vi "DISP_WIND_TRAC_FEED.vi"(0 "VISA IN":refnum<visa-resource-name>, 1 "Trace":i32=1, 2 "Name":string, 5 "error in":errorcluster, 7 "Window":i32=1) -> (14 "VISA Out":refnum<visa-resource-name>, 19 "error out":errorcluster)   [LabVIEW 2018, in "PNA-X.lvlib"]
doc: "DISPlay:WINDow<wnum>:TRACe<tnum>:FEED <name> \n1595\n\n(Write-only) Creates a new trace <tnum> and associates (feeds) a measurement <name> to the \nspecified window<wnum>. This command should be executed immediately after creating a new \nmeasurement with CALC:PAR:DEF<name>,<parameter>. \nTo feed the same measurement to multiple traces, create another measurement with the same \n<name>,<parameter> using the CALC:PAR:DEF command. The analyzer will collect the data only \nonce. \nParameters \n<wnum> Any existing window number. If unspecified, value is set to 1. \n<tnum> Trace number to be created. Choose any Integer between 1 and 8 \n<name> Name of the measurement that was defined with \nCALC:PAR:DEF<name>,<parameter> \nExamples DISP:WIND:TRAC:FEED 'test' \ndisplay:window2:trace2:feed 'test' \nQuery Syntax Not applicable \nDefault \"CH1_S11\""
uses:
  PNA-X.lvlib
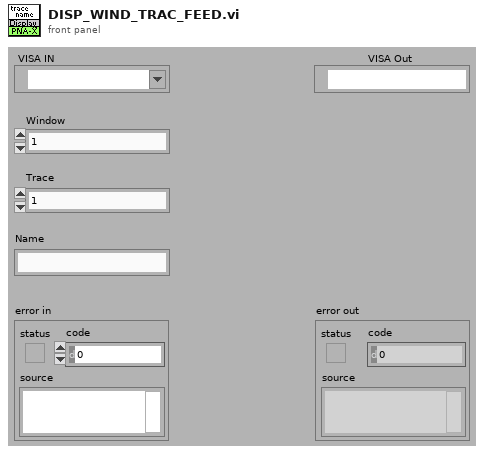
[diagram p1: front panel]
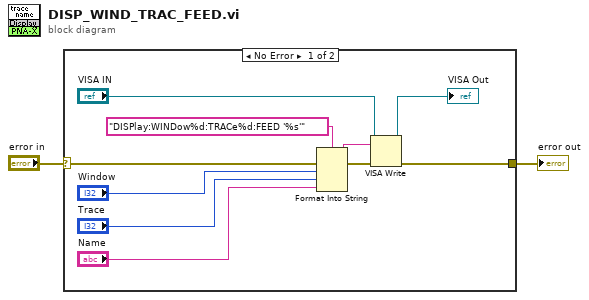
[diagram p0: block diagram]
diagram:
  n1 = case shown="No Error" "error in" {
    selector: "error in" -> [w12 w13]
    tunnel: [w7 w13] -> w1
    frame No Error {
      n2 = Format Into String(format string="DISPlay:WINDow%d:TRACe%d:FEED '%s'" ("Cmdline"), error in=w12, "Window", "Trace", "Name") -> (resulting string=w10:string, error out=w11:errorcluster)  [unwired: 1 in]
      n3 = VISA Write(VISA resource name="VISA IN", write buffer=w10, error in (no error)=w11) -> (VISA resource name out=→"VISA Out":refnum<visa-resource-name>, error out=w7:errorcluster)  [unwired: 1 out]
    }
    frame Error {
    }
  }
  "error out" <- w1
